vi "grid_and_guides.vi"(9 "Boolean":bool, 10 "Operation":T2(ring), 11 "Image":T1) -> (3 "Image Out":T1)   [LabVIEW 2010]
doc: "This sets up where the grid and guides go.\n\n(the line below ensures settings are saved)\n[Red Tweezers Save Settings]"
uses:
  <vilib>/vision/Image Controls.llb/IMAQ Image.ctl
panel:
  in  "Tab Control":enum32{"Guides", "Grid"}(tab)
  in  "Guides":T3(array[cluster])
  in  "Show Guides":bool
  in  "Show Grid":bool
  in  "Grid Spacing":dbl
  # "just close this window when you are done"
  # "You can set up guides here, which will appear on the image.  They can be turned on and off from the \"view\" menu"
  # "You can have a grid of regularly spaced guides across the sample, which is used by the \"snap to grid\" function of the \"current spot\" tab."
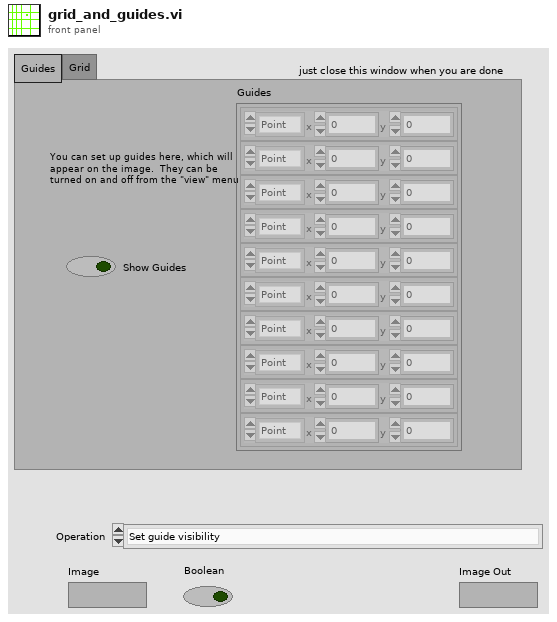
[diagram p1: front panel]
types:
  T1 = typedef "IMAQ Image.ctl" = refnum<image>
  T2 = enum16{"Set guide visibility", "Set grid visibility", "Show front panel", "Render on image"}
  T3 = cluster{"Enum":enum16{"Point", "Cross", "Vertical", "Horizontal"}, "x":dbl, "y":dbl}[]
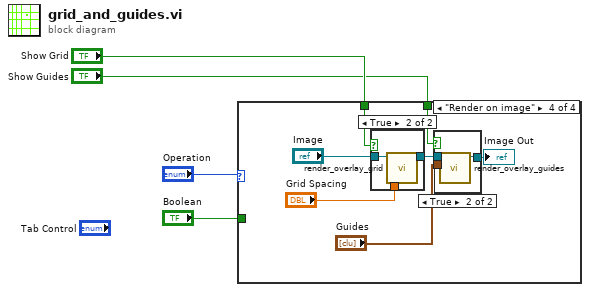
[diagram p0: block diagram]
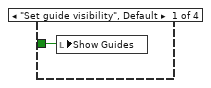
[diagram p2: hidden frame]
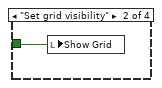
[diagram p3: hidden frame]
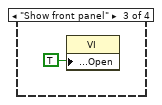
[diagram p4: hidden frame]
diagram:
  n1 = case shown="\"Render on image\"" "Operation" {
    tunnel: "Boolean" -> [w5 w6 _ _]
    tunnel: "Show Grid" -> [_ _ _ w9]
    tunnel: "Show Guides" -> [_ _ _ w8]
    frame "Set guide visibility", Default {
      n2 = local write "Show Guides"(w5) -> ()
    }
    frame "Set grid visibility" {
      n3 = local write "Show Grid"(w6) -> ()
    }
    frame "Show front panel" {
      n4 = property class="VI"("Front Panel.Open"=TRUE ("Front Panel Window:Open")) -> ()  [unwired: 2 in, 2 out]
    }
    frame "Render on image" {
      n5 = case shown="True" w9 {
        tunnel: "Grid Spacing" -> [_ w22]
        tunnel: "Image" -> [w19 w21]
        tunnel: [w19 w20] -> w11
        frame False {
        }
        frame True {
          n6 = call "render_overlay_grid.vi"("Grid Spacing"=w22, "Image"=w21) -> ("Image Out"=w20:T1)  [unwired: 5 in]
        }
      }
      n7 = case shown="True" w8 {
        tunnel: "Guides" -> [_ w18]
        tunnel: w11 -> [w15 w17]
        tunnel: [w15 w16] -> w10
        frame False {
        }
        frame True {
          n8 = call "render_overlay_guides.vi"("Guides"=w18, "Image Out 2"=w17) -> ("Image Out"=w16:T1)  [unwired: 5 in]
        }
      }
      "Image Out" <- w10
    }
  }
